vi "Load Configuration From File.vi"(8 "error in (no error)":errorcluster, 9 "Instance Name":string, 10 "Configuration Path":path, 11 "Xbox Controller-Physical in":refnum<class "Xbox Controller-Physical.lvclass">) -> (0 "error out":errorcluster, 3 "Xbox Controller-Physical out":refnum<class "Xbox Controller-Physical.lvclass">)   [LabVIEW 2013, in "Physical Systems.lvlib" / "XBox Controller.lvlib" / "Xbox Controller-Physical.lvclass"]
uses:
  Xbox Controller-Physical.lvclass
  Virtual Systems/XBox Controller/XBox Controller Class/XBox Controller-Logical.lvclass
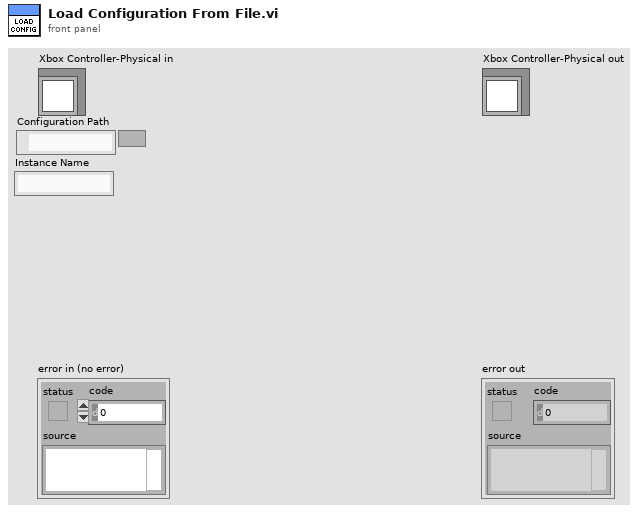
[diagram p1: front panel]
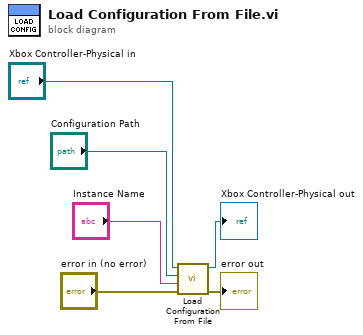
[diagram p0: block diagram]
diagram:
  n1 = call-parent "Load Configuration From File.vi"("error in (no error)"="error in (no error)", "Instance Name"="Instance Name", "Configuration Path"="Configuration Path", "System Actor in"="Xbox Controller-Physical in") -> ("error out"=→"error out":errorcluster, "System Actor out"=→"Xbox Controller-Physical out":refnum<class "Xbox Controller-Physical.lvclass">)  [unwired: 6 in]
